vi "Car_barrier.vi"() -> ()   [LabVIEW 2020]
panel:
  in  "DCY":bool
  in  "BP2":bool
  in  "BP1":bool
  out "RED":bool
  out "GREEN":bool
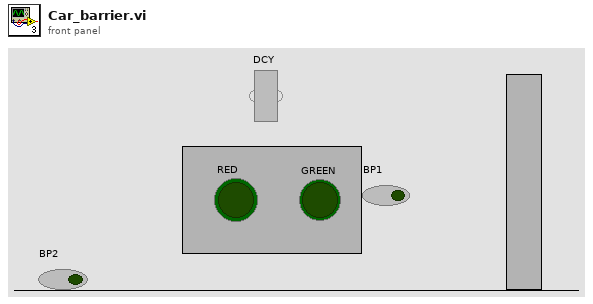
[diagram p1: front panel]
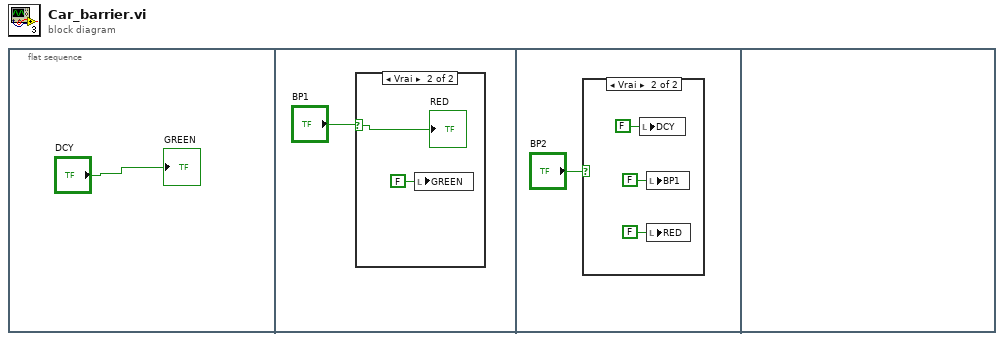
[diagram p0: block diagram]
diagram:
  n1 = flat-sequence {
    frame #0 {
      "GREEN" <- "DCY"
    }
    frame #1 {
      n2 = case shown="Vrai" "BP1" {
        selector: "BP1" -> [_ w4]
        frame False {
        }
        frame True {
          n3 = local write "GREEN"(FALSE ("GREEN")) -> ()
          "RED" <- w4
        }
      }
    }
    frame #2 {
      n4 = case shown="Vrai" "BP2" {
        frame False {
        }
        frame True {
          n5 = local write "DCY"(FALSE ("DCY")) -> ()
          n6 = local write "BP1"(FALSE ("BP1")) -> ()
          n7 = local write "RED"(FALSE ("RED")) -> ()
        }
      }
    }
    frame #3 {
    }
  }
